vi "GetFlattenedString.vi"(8 "error in":errorcluster, 11 "Integer in":refnum<class "Integer.lvclass">) -> (0 "error out":errorcluster, 2 "FlattenedString":string, 3 "Integer out":refnum<class "Integer.lvclass">)   [LabVIEW 2021, in "ProligentXMLGenerator.lvlib" / "Integer.lvclass"]
uses:
  Integer.lvclass
  Integer.lvclass/Integer.ctl
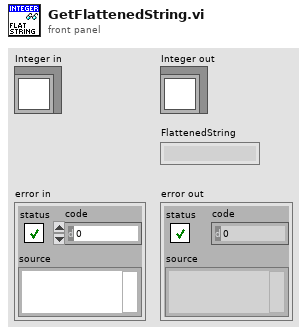
[diagram p1: front panel]
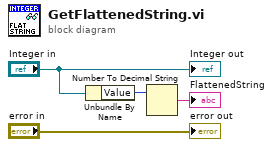
[diagram p0: block diagram]
diagram:
  n1 = Unbundle By Name("Integer in") -> ("Value"=w1:i64)
  n2 = Number To Decimal String(number=w1) -> (decimal integer string=→"FlattenedString":string)  [unwired: 1 in]
  "error out" <- "error in"
  "Integer out" <- "Integer in"
